vi "toml_api.vi"(7 "cmd":string, 8 "error in (no error)":errorcluster, 10 "data in":variant, 11 "resolved path":path) -> (0 "error out":errorcluster, 1 "exists":bool, 2 "data out":variant, 3 "files":path[](array[path]))   [LabVIEW 2017]
uses:
  <vilib>/Utility/libraryn.llb/Check if File or Folder Exists.vi
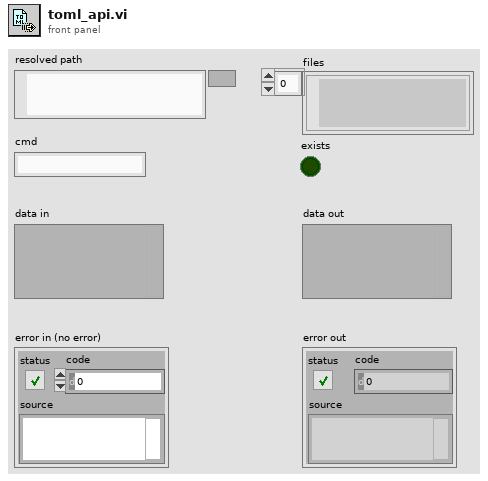
[diagram p1: front panel]
types:
  T1 = enum16{"open", "replace", "create", "open or create", "replace or create", "replace or create with confirmation"}
  T2 = cluster{"section":string, "key":string, "value":variant}
  T3 = cluster{"s":string, "#":string, "..":string, "kv#p":string[][]}[]
  T4 = cluster{"s":string, "#":string, "..":string, "kv#p":string[][]}
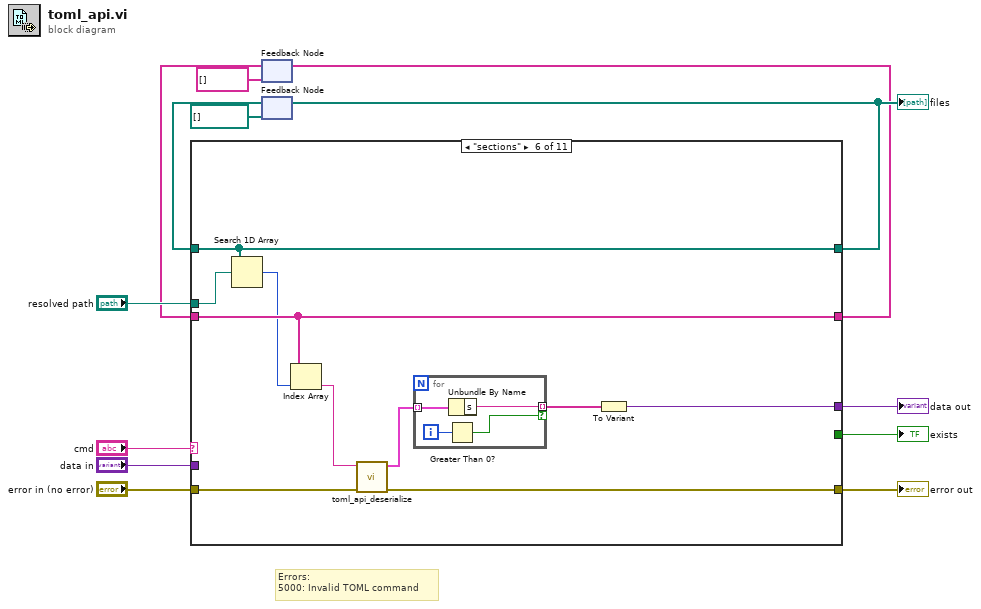
[diagram p0: block diagram]
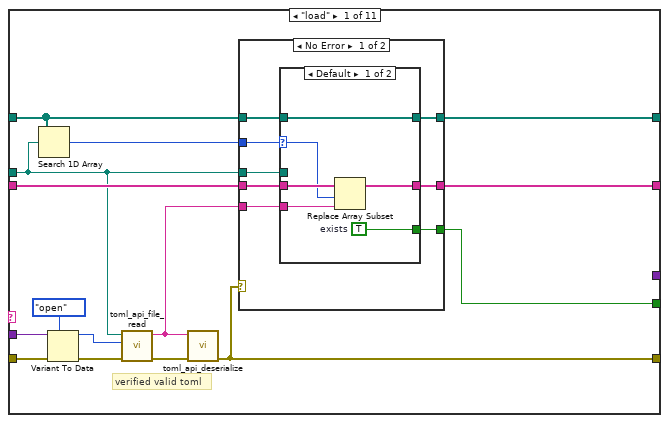
[diagram p2: hidden frame]
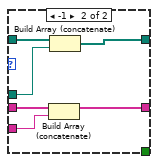
[diagram p3: hidden frame]
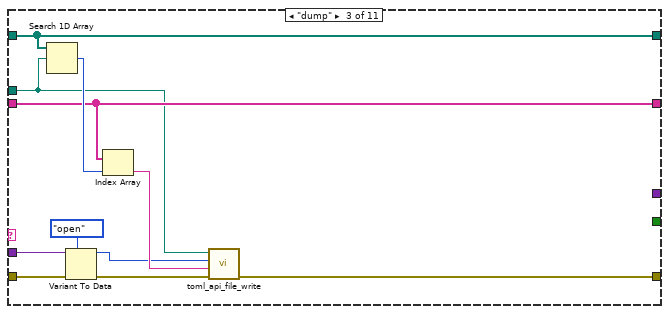
[diagram p6: hidden frame]
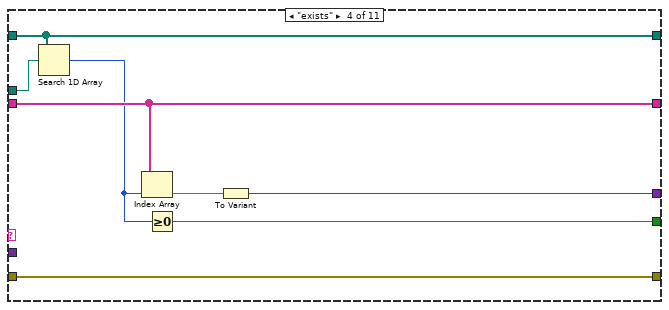
[diagram p7: hidden frame]
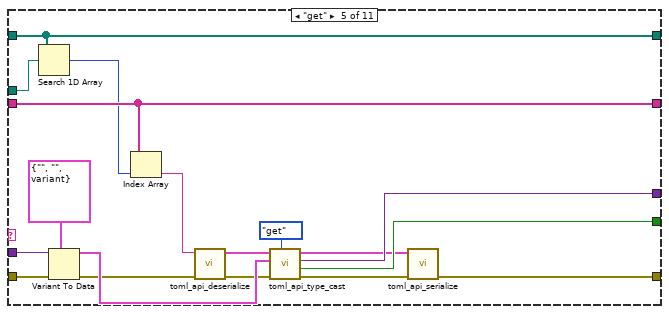
[diagram p8: hidden frame]
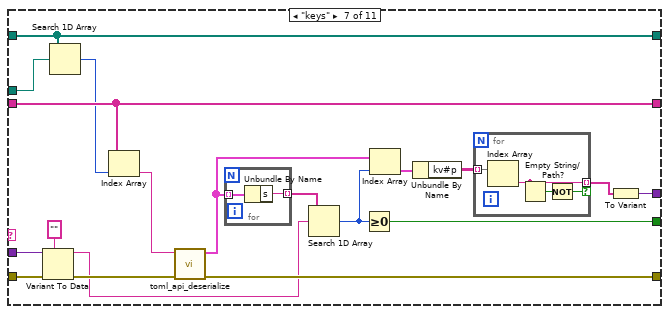
[diagram p9: hidden frame]
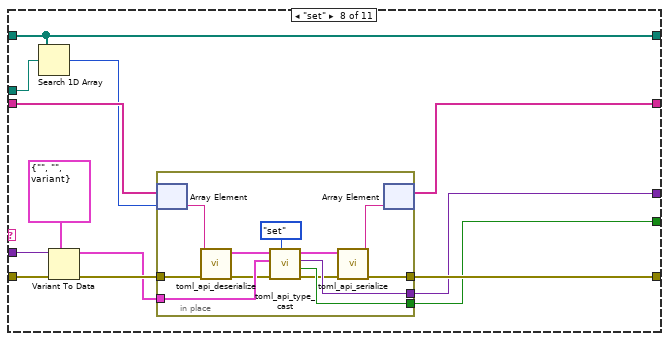
[diagram p10: hidden frame]
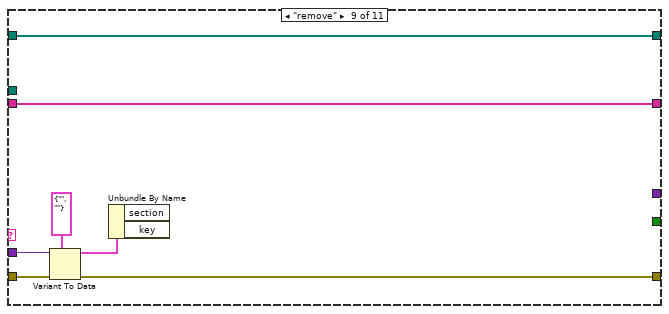
[diagram p11: hidden frame]
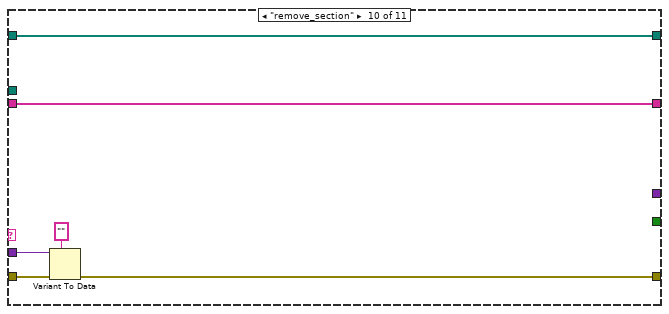
[diagram p12: hidden frame]
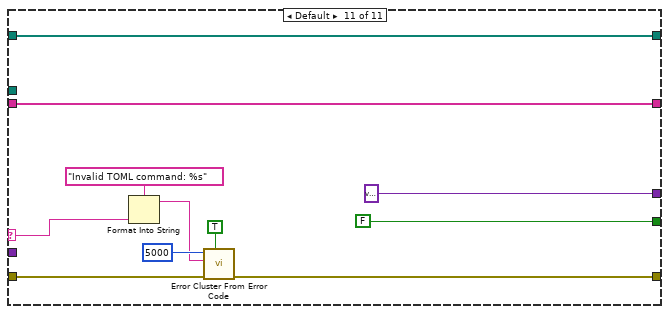
[diagram p13: hidden frame]
diagram:
  # "Errors:\n5000: Invalid TOML command"
  n1 = feedback #1(string[] []) -> (w4:string[])
  n2 = feedback #2(path[] []) -> (w8:path[])
  n3 = case shown="\"sections\"" "cmd" {
    selector: "cmd" -> [_ _ _ _ _ _ _ _ _ _ w170]
    tunnel: [w14 w53 w60 w70 w78 w94 w117 w136 w160 w166 w173] -> w12
    tunnel: "error in (no error)" -> [w25 w53 w61 w70 w88 w95 w118 w140 w161 w167 w174]
    tunnel: "resolved path" -> [w19 _ w59 w71 w89 w99 w122 w141 _ _ _]
    tunnel: w8 -> [w28 w52 w64 w72 w90 w100 w123 w142 w156 w164 w177]
    tunnel: [w21 w52 w64 w72 w90 w100 w123 w142 w156 w164 w177] -> w7
    tunnel: [w26 w51 w62 w68 w87 w98 w121 w130 w155 w163 w178] -> w5
    tunnel: w4 -> [w27 w51 w62 w68 w87 w98 w121 w132 w155 w163 w178]
    tunnel: "data in" -> [w24 _ w56 _ w85 _ w113 w139 w159 w165 _]
    tunnel: [_ _ _ w65 w82 w96 w119 w134 _ _ variant] -> w2
    tunnel: [w18 _ _ w69 w81 _ w108 w133 _ _ FALSE] -> w1
    frame "load" {
      # "verified valid toml"
      n4 = Search 1D Array(1D array=w28, element=w19) -> (index of element=w20:i32)  [unwired: 1 in]
      n5 = Variant To Data(error in=w25, type=T1."open" ("operation"), Variant=w24) -> (data=w22:T1, error out=w23:errorcluster)
      n6 = call "toml_api_file_read.vi"("error in (no error)"=w23, "operation (open or create)"=w22, "resolved path"=w19) -> ("error out"=w16:errorcluster, "text"=w15:string)  [unwired: 7 in]
      n7 = call "toml_api_deserialize.vi"("error in (no error)"=w16, "text in"=w15) -> ("error out"=w14:errorcluster)  [unwired: 8 in, 1 out]
      n8 = case shown="No Error" w14 {
        tunnel: w28 -> [w36 w50]
        tunnel: w27 -> [w35 w49]
        tunnel: [w34 w49] -> w26
        tunnel: [w33 w50] -> w21
        tunnel: w20 -> [w32 _]
        tunnel: w19 -> [w31 _]
        tunnel: [w30 _] -> w18
        tunnel: w15 -> [w29 _]
        frame No Error {
          n9 = case shown="Default" w32 {
            selector: w32 -> [w37 _]
            tunnel: w36 -> [w42 w48]
            tunnel: w35 -> [w41 w47]
            tunnel: [w40 w46] -> w34
            tunnel: w29 -> [w39 w45]
            tunnel: [w42 w44] -> w33
            tunnel: w31 -> [_ w43]
            tunnel: [w38 _] -> w30
            frame Default {
              w38 = TRUE  # exists
              n10 = Replace Array Subset(array=w41, new element=w39, index=w37) -> (w40:string[])
            }
            frame -1 {
              n11 = Build Array (concatenate)(w47, w45) -> (w46:string[])
              n12 = Build Array (concatenate)(w48, w43) -> (w44:path[])
            }
          }
        }
        frame Error {
        }
      }
    }
    frame "null" {
    }
    frame "dump" {
      n13 = Search 1D Array(1D array=w64, element=w59) -> (index of element=w63:i32)  [unwired: 1 in]
      n14 = Variant To Data(error in=w61, type=T1."open" ("operation (replace or create)"), Variant=w56) -> (data=w54:T1, error out=w57:errorcluster)
      n15 = Index Array(array=w62, index=w63) -> (element=w58:string)
      n16 = call "toml_api_file_write.vi"("error in (no error)"=w57, "text"=w58, "operation (replace or create)"=w54, "resolved path"=w59) -> ("error out"=w60:errorcluster)  [unwired: 7 in]
    }
    frame "exists" {
      n17 = Search 1D Array(1D array=w72, element=w71) -> (index of element=w67:i32)  [unwired: 1 in]
      n18 = Index Array(array=w68, index=w67) -> (element=w66:string)
      n19 = Greater Or Equal To 0?(x=w67) -> (x >= 0?=w69:bool)
      n20 = To Variant(anything=w66) -> (Variant=w65:variant)
    }
    frame "get" {
      n21 = Search 1D Array(1D array=w90, element=w89) -> (index of element=w86:i32)  [unwired: 1 in]
      n22 = Variant To Data(error in=w88, type=T2 {"section"="", "key"="", "value"=variant} ("item"), Variant=w85) -> (data=w80:T2, error out=w76:errorcluster)
      n23 = Index Array(array=w87, index=w86) -> (element=w74:string)
      n24 = call "toml_api_deserialize.vi"("error in (no error)"=w76, "text in"=w74) -> ("error out"=w75:errorcluster, "sections"=w73:T3)  [unwired: 8 in]
      n25 = call "toml_api_type_cast.vi"("action"=enum8{"get", "set"}."get", "error in (no error)"=w75, "item"=w80, "sections in"=w73) -> ("error out"=w79:errorcluster, "exists?"=w81:bool, "value"=w82:variant, "sections out"=w77:T3)  [unwired: 4 in]
      n26 = call "toml_api_serialize.vi"("error in (no error)"=w79, "sections"=w77) -> ("error out"=w78:errorcluster)  [unwired: 8 in, 1 out]
    }
    frame "sections" {
      n27 = Search 1D Array(1D array=w100, element=w99) -> (index of element=w97:i32)  [unwired: 1 in]
      n28 = Index Array(array=w98, index=w97) -> (element=w93:string)
      n29 = call "toml_api_deserialize.vi"("error in (no error)"=w95, "text in"=w93) -> ("error out"=w94:errorcluster, "sections"=w92:T3)  [unwired: 8 in]
      n30 = for {
        tunnel: w92 -> [w104] mode=indexing
        tunnel: [w103] -> w91 mode=indexing if=w101
        i -> [w102]
        n31 = Greater Than 0?(x=w102) -> (x > 0?=w101:bool)
        n32 = Unbundle By Name(w104) -> ("s"=w103:string)
      }
      n33 = To Variant(anything=w91) -> (Variant=w96:variant)
    }
    frame "keys" {
      n34 = Variant To Data(error in=w118, type="", Variant=w113) -> (data=w111:string, error out=w114:errorcluster)
      n35 = Search 1D Array(1D array=w123, element=w122) -> (index of element=w120:i32)  [unwired: 1 in]
      n36 = Index Array(array=w121, index=w120) -> (element=w116:string)
      n37 = call "toml_api_deserialize.vi"("error in (no error)"=w114, "text in"=w116) -> ("error out"=w117:errorcluster, "sections"=w110:T3)  [unwired: 8 in]
      n38 = for {
        tunnel: w110 -> [w129] mode=indexing
        tunnel: [w128] -> w115 mode=indexing
        n39 = Unbundle By Name(w129) -> ("s"=w128:string)
      }
      n40 = Search 1D Array(1D array=w115, element=w111) -> (index of element=w109:i32)  [unwired: 1 in]
      n41 = Greater Or Equal To 0?(x=w109) -> (x >= 0?=w108:bool)
      n42 = Index Array(array=w110, index=w109) -> (element=w107:T4)
      n43 = Unbundle By Name(w107) -> ("kv#p"=w106:string[][])
      n44 = for {
        tunnel: w106 -> [w127] mode=indexing
        tunnel: [w126] -> w105 mode=indexing if=w124
        n45 = Index Array(array=w127) -> (element=w126:string)  [unwired: 1 in]
        n46 = Empty String/Path?(string/path=w126) -> (empty?=w125:bool)
        n47 = Not(x=w125) -> (.not. x?=w124:bool)
      }
      n48 = To Variant(anything=w105) -> (Variant=w119:variant)
    }
    frame "set" {
      n49 = Search 1D Array(1D array=w142, element=w141) -> (index of element=w131:i32)  [unwired: 1 in]
      n50 = Variant To Data(error in=w140, type=T2 {"section"="", "key"="", "value"=variant} ("item"), Variant=w139) -> (data=w135:T2, error out=w137:errorcluster)
      n51 = in-place {
        in-place-border: w137 -> [w150]
        in-place-border: [w145] -> w136
        in-place-border: w135 -> [w154]
        in-place-border: [w152] -> w134
        in-place-border: [w151] -> w133
        n52 = in-place-array #3(w132, w131) -> (w148:string)
        n53 = call "toml_api_deserialize.vi"("error in (no error)"=w150, "text in"=w148) -> ("error out"=w149:errorcluster, "sections"=w147:T3)  [unwired: 8 in]
        n54 = call "toml_api_type_cast.vi"("action"=enum8{"get", "set"}."set", "error in (no error)"=w149, "item"=w154, "sections in"=w147) -> ("error out"=w146:errorcluster, "exists?"=w151:bool, "value"=w152:variant, "sections out"=w144:T3)  [unwired: 4 in]
        n55 = call "toml_api_serialize.vi"("error in (no error)"=w146, "sections"=w144) -> ("error out"=w145:errorcluster, "text out"=w143:string)  [unwired: 8 in]
        n56 = in-place-array #3(w143) -> (w130:string[])  [unwired: 1 out]
      }
    }
    frame "remove" {
      n57 = Variant To Data(error in=w161, type=cluster{"section":string, "key":string} {"section"="", "key"=""} ("cluster"), Variant=w159) -> (data=w157:cluster{"section":string, "key":string}, error out=w160:errorcluster)
      n58 = Unbundle By Name(w157) -> ()  [unwired: 2 out]
    }
    frame "remove_section" {
      n59 = Variant To Data(error in=w167, type="" ("section"), Variant=w165) -> (error out=w166:errorcluster)  [unwired: 1 out]
    }
    frame Default {
      n60 = Format Into String(format string="Invalid TOML command: %s" ("error message (\"\")"), w170) -> (resulting string=w168:string)  [unwired: 2 in, 1 out]
      n61 = call <vilib>:"Error Cluster From Error Code.vi"("show call chain? (False)"=TRUE, "error in (no error)"=w174, "error message (\"\")"=w168, "error code (0)"=5000) -> ("error out"=w173:errorcluster)  [unwired: 5 in]
    }
  }
  "error out" <- w12
  "data out" <- w2
  "files" <- w7
  "exists" <- w1
  n62 = feedback-in #1(w5) -> ()
  n63 = feedback-in #2(w7) -> ()
